vi "Read Stable Cond.vi"(8 "error in (no error)":errorcluster, 11 "DeepU Results in":refnum<class "DeepU Results.lvclass">) -> (0 "error out":errorcluster, 2 "Stable Cond":bool caption="Stable Conditions", 3 "DeepU Results out":refnum<class "DeepU Results.lvclass">)   [LabVIEW 2019, in "Results.lvlib" / "DeepU Results.lvclass"]
uses:
  DeepU Results.lvclass
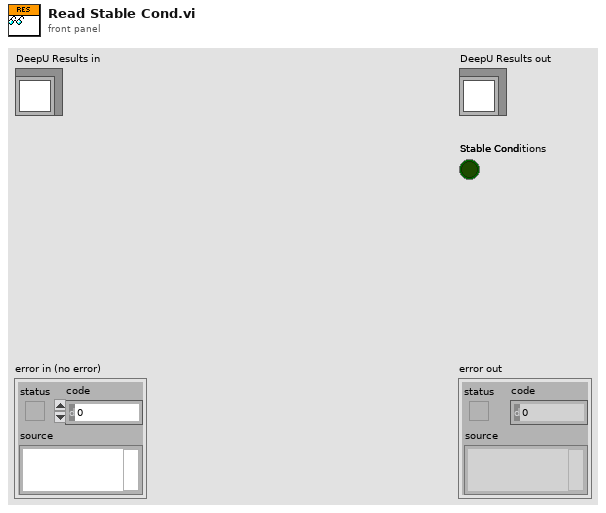
[diagram p1: front panel]
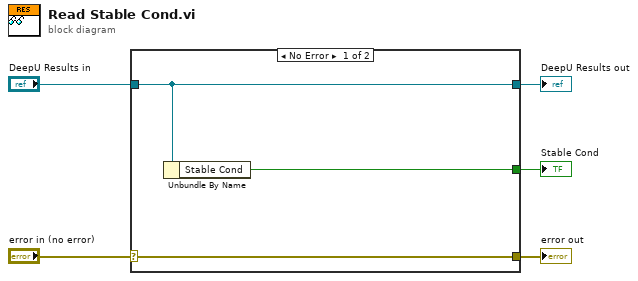
[diagram p0: block diagram]
diagram:
  n1 = case shown="No Error" "error in (no error)" {
    selector: "error in (no error)" -> [w8 w9]
    tunnel: [w8 w9] -> w4
    tunnel: [w7 w10] -> w2
    tunnel: "DeepU Results in" -> [w7 w10]
    tunnel: [w6 _] -> w1
    frame No Error {
      n2 = Unbundle By Name(w7) -> ("Stable Cond"=w6:bool)
    }
    frame Error {
    }
  }
  "error out" <- w4
  "DeepU Results out" <- w2
  "Stable Cond" <- w1
